vi "addNewTable.vi"(8 "error in (no error)":errorcluster, 10 "New Paragraph":refnum<class "xwpfTable.lvclass">, 11 "xwpfDocument in":refnum<class "xwpfDocument.lvclass">) -> (0 "error out":errorcluster, 3 "xwpfDocument out":refnum<class "xwpfDocument.lvclass">)   [LabVIEW 2017, in "Word_Specific.lvlib" / "xwpfDocument.lvclass"]
uses:
  xwpfDocument.lvclass
  xwpfTable/xwpfTable.lvclass
  xwpfDocument.lvclass/xwpfDocument.ctl
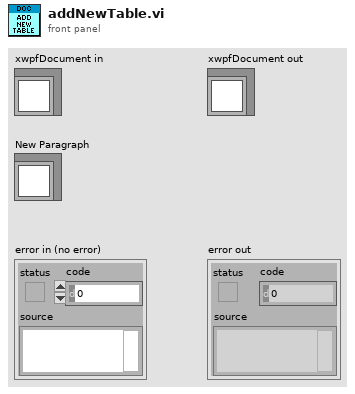
[diagram p1: front panel]
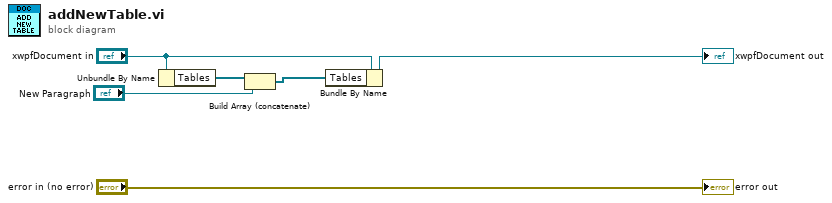
[diagram p0: block diagram]
diagram:
  n1 = Unbundle By Name("xwpfDocument in") -> ("Tables"=w4:refnum<class "xwpfTable.lvclass">[])
  n2 = Build Array (concatenate)(w4, "New Paragraph") -> (w3:refnum<class "xwpfTable.lvclass">[])
  n3 = Bundle By Name(cluster="xwpfDocument in", "Tables"=w3) -> (→"xwpfDocument out":refnum<class "xwpfDocument.lvclass">)
  "error out" <- "error in (no error)"
